vi "wykresy rejestracja_opis.vi"(8 "error in (no error)":errorcluster, 11 "Wykres Ref in":refnum<vi>) -> (0 "error out":errorcluster)   [LabVIEW 2014]
doc: "Przypisuje nazwy i zmienia skale wykresów w zakładce Rejestracja"
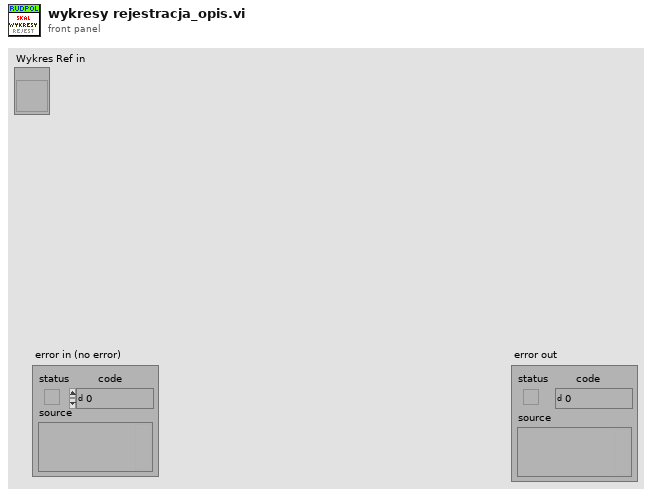
[diagram p1: front panel]
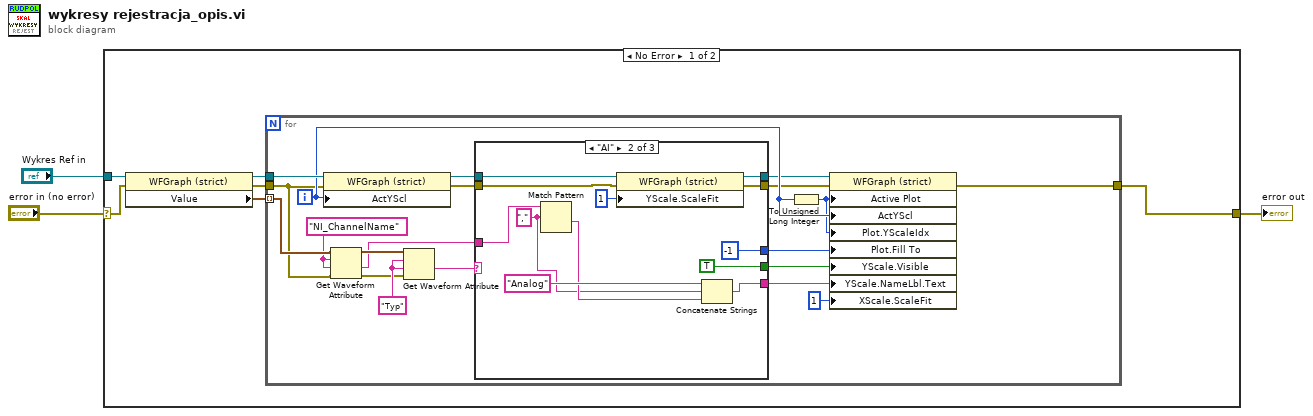
[diagram p0: block diagram]
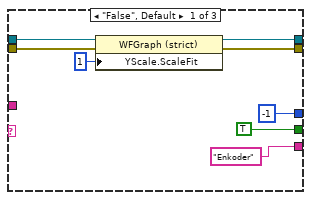
[diagram p2: hidden frame]
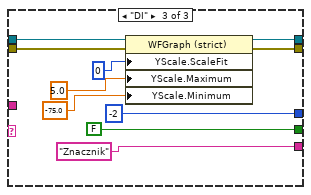
[diagram p3: hidden frame]
diagram:
  n1 = case shown="No Error" "error in (no error)" {
    selector: "error in (no error)" -> [w8 w60]
    tunnel: [w4 w60] -> w2
    tunnel: "Wykres Ref in" -> [w9 _]
    frame No Error {
      n2 = property class="WFGraph (strict)"(reference=w9, error in=w8) -> (reference out=w7:refnum<vi>, error out=w5:errorcluster, "Value"=w6:waveform(dbl)[])
      n3 = for {
        tunnel: w7 -> [w29]
        tunnel: w6 -> [w18] mode=indexing
        tunnel: w5 -> [w17]
        tunnel: [w21] -> w4
        i -> [w26]
        w14 = "NI_ChannelName" ("name")
        w27 = "Typ" ("name")
        n4 = property class="WFGraph (strict)"(reference=w29, error in=w17, "ActYScl"=w26) -> (reference out=w11:refnum<vi>, error out=w28:errorcluster)
        n5 = Get Waveform Attribute(4:w17, 5:w14, 6:w14, 7:w18) -> (0:w16:errorcluster, 1:w13:string, 3:w15:waveform(dbl))  [unwired: 1 out]
        n6 = Get Waveform Attribute(4:w16, 5:w27, 6:w27, 7:w15) -> (1:w20:string)  [unwired: 3 out]
        n7 = case shown="\"AI\"" w20 {
          tunnel: w11 -> [w32 w41 w55]
          tunnel: w28 -> [w33 w40 w56]
          tunnel: [i16 -1 ("Plot.Fill To") i16 -1 ("Plot.Fill To") i16 -2 ("Plot.Fill To")] -> w24
          tunnel: [TRUE ("Y Scale.Visible") TRUE ("Y Scale.Visible") FALSE ("Y Scale.Visible")] -> w23
          tunnel: [w31 w39 w54] -> w22
          tunnel: ["Enkoder" ("name") w46 "Znacznik" ("name")] -> w19
          tunnel: w13 -> [_ w47 _]
          tunnel: [w30 w38 w53] -> w10
          frame "False", Default {
            n8 = property class="WFGraph (strict)"(reference=w32, error in=w33, "YScale.ScaleFit"=u8 1 ("Y Scale.Scale Fit")) -> (reference out=w30:refnum<vi>, error out=w31:errorcluster)
          }
          frame "AI" {
            w43 = "," ("regular expression")
            n9 = Match Pattern(string=w47, regular expression=w43) -> (after substring=w44:string)  [unwired: 1 in, 3 out]
            n10 = property class="WFGraph (strict)"(reference=w41, error in=w40, "YScale.ScaleFit"=u8 1 ("Y Scale.Scale Fit")) -> (reference out=w38:refnum<vi>, error out=w39:errorcluster)
            n11 = Concatenate Strings("Analog" ("name"), w43, w44) -> (w46:string)
          }
          frame "DI" {
            n12 = property class="WFGraph (strict)"(reference=w55, error in=w56, "YScale.ScaleFit"=u8 0 ("X Scale.Scale Fit"), "YScale.Maximum"=5.0 ("Y Scale.Range:Maximum"), "YScale.Minimum"=-75.0 ("Y Scale.Range:Minimum")) -> (reference out=w53:refnum<vi>, error out=w54:errorcluster)
          }
        }
        n13 = To Unsigned Long Integer(number=w26) -> (unsigned 32bit integer=w25:u32)
        n14 = property class="WFGraph (strict)"(reference=w10, error in=w22, "Active Plot"=w25, "ActYScl"=w26, "Plot.YScaleIdx"=w25, "Plot.Fill To"=w24, "YScale.Visible"=w23, "YScale.NameLbl.Text"=w19, "XScale.ScaleFit"=u8 1 ("X Scale.Scale Fit")) -> (error out=w21:errorcluster)  [unwired: 1 out]
      }
    }
    frame Error {
    }
  }
  "error out" <- w2
